vi "Launcher (Top Level).vi"(8 "error in":errorcluster) -> (0 "error out":errorcluster)   [LabVIEW 2010]
doc: "This VI is the launcher for the ATM Simulator.\n\nThis VI performs any actions required to occur before the modules begin running or after they close (such as creating the user events). It then launches the modules. The UI is launched dynamically when the program is run. \n\n[Covers: SI1]\n[Covers: SI2]"
uses:
  User Events/Controls/UE Abort Action.ctl
  Modules/Error Handler/Error Handler.lvlib
  Modules/Simulated Console (UI)/Simulated Console.lvlib
  Modules/Controller/Contoller.lvlib
  Modules/Config DataBase/Config Database.lvlib
  Modules/Sensor/Sensor Console/Sensor Console.lvlib
  Modules/Display/Display Console/Display Console.lvlib
panel:
  # "This VI is the launcher for the ATM Simulator.\n\nThis VI performs any actions required to occur before the modules begin running or after they close \n(such as creating the user events). \nIt then launches the modules. The UI is launched dynamically when the program is run."
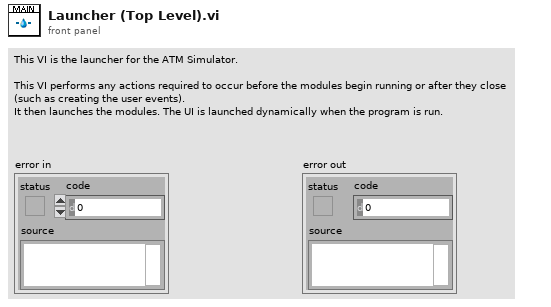
[diagram p1: front panel]
types:
  T1 = typedef "UE Abort Action.ctl" = enum16{"Destroy", "Get", "Create"}
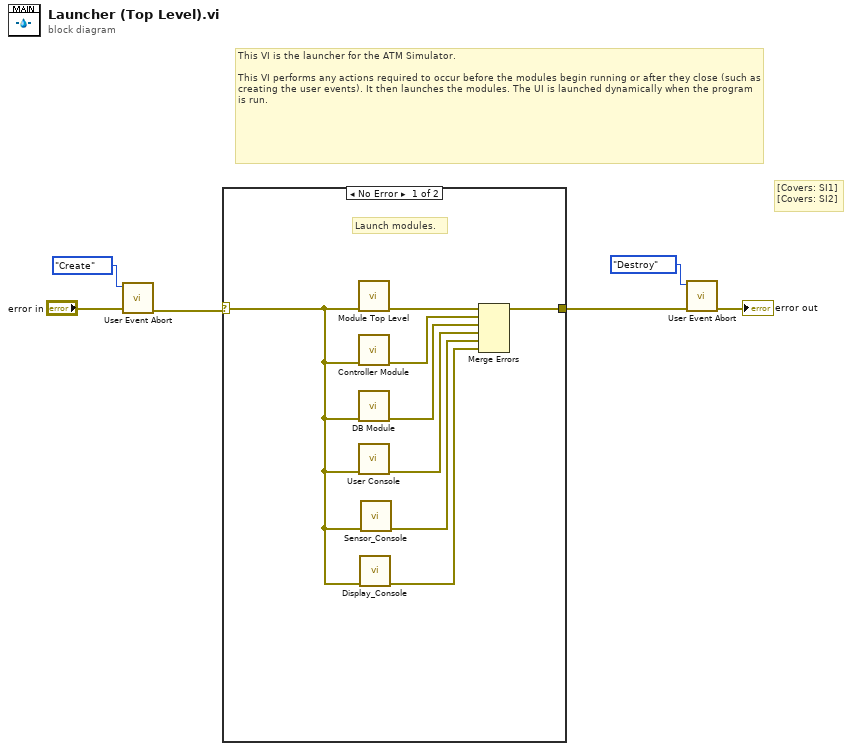
[diagram p0: block diagram]
diagram:
  # "[Covers: SI1]\n[Covers: SI2]"
  # "This VI is the launcher for the ATM Simulator.\n\nThis VI performs any actions required to occur before the modules begin running or after they close (such as creating the user events). It then launches the modules. The UI is launched dynamically when the program is run."
  n1 = call "User Event Abort.vi"("error in"="error in", "Action"=UE_Abort_Action."Create") -> ("error out"=w5:errorcluster)  [unwired: 8 in, 1 out]
  n2 = case shown="No Error" w5 {
    selector: w5 -> [w7 w15]
    tunnel: [w10 w15] -> w2
    frame No Error {
      # "Launch modules."
      n3 = call "Module Top Level.vi"("error in"=w7) -> ("error out"=w14:errorcluster)  [unwired: 10 in]
      n4 = call "Controller Module.vi"("error in"=w7) -> ("error out"=w13:errorcluster)  [unwired: 10 in]
      n5 = call "DB Module.vi"("error in"=w7) -> ("error out"=w12:errorcluster)  [unwired: 10 in]
      n6 = call "User Console.vi"("error in"=w7) -> ("error out"=w11:errorcluster)  [unwired: 10 in]
      n7 = call "Display_Console.vi"("error in"=w7) -> ("error out"=w8:errorcluster)  [unwired: 10 in]
      n8 = call "Sensor_Console.vi"("error in"=w7) -> ("error out"=w9:errorcluster)  [unwired: 10 in]
      n9 = Merge Errors(w14, w13, w12, w11, w9, w8) -> (w10:errorcluster)
    }
    frame Error {
      # "Handle error and do not launch."
    }
  }
  n10 = call "User Event Abort.vi"("error in"=w2, "Action"=UE_Abort_Action."Destroy") -> ("error out"=→"error out":errorcluster)  [unwired: 8 in, 1 out]
